vi "Single Shimmer.vi"() -> ()   [LabVIEW 2025]
uses:
  C:/Github/Shimmer-Labview-API/ShimmerLabview/Bin/ShimmerLVWrapper.dll
  Bin/ShimmerLVWrapper.dll
panel:
  out "Waveform Chart":cluster{dbl, dbl, dbl}(graph)
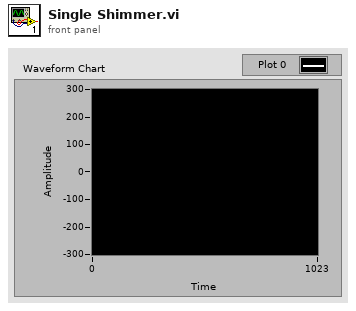
[diagram p1: front panel]
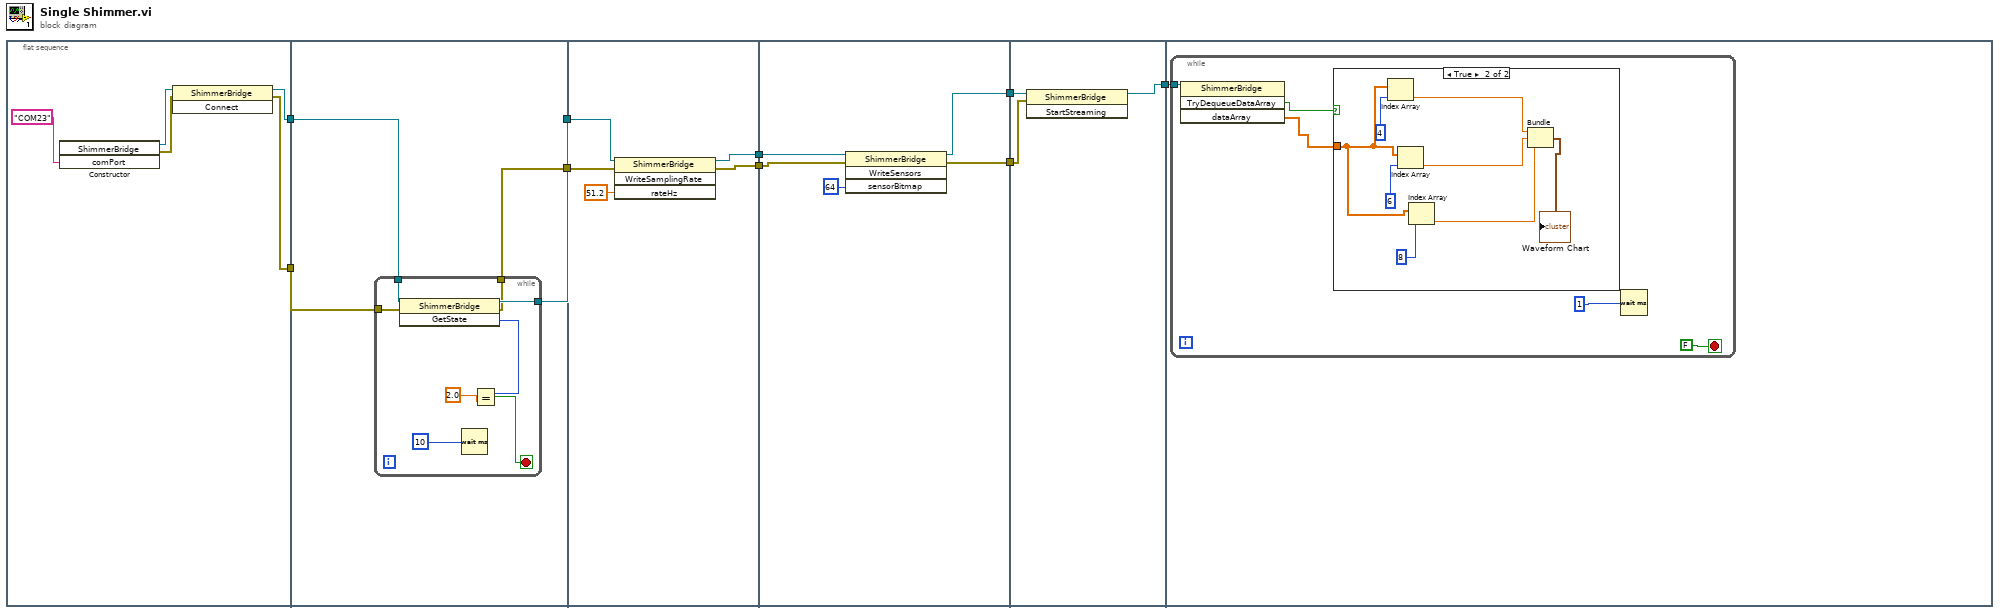
[diagram p0: block diagram]
diagram:
  n1 = flat-sequence {
    tunnel: [w11] -> w9
    tunnel: [w10] -> w4
    tunnel: w9 -> [w18]
    tunnel: [w17] -> w7
    tunnel: w4 -> [w15]
    tunnel: [w16] -> w1
    tunnel: w7 -> [w31]
    tunnel: [w30] -> w6
    tunnel: [w29] -> w3
    tunnel: w1 -> [w27]
    tunnel: w6 -> [w36]
    tunnel: [w35] -> w5
    tunnel: w3 -> [w34]
    tunnel: [w33] -> w2
    tunnel: [w39] -> w8
    tunnel: w5 -> [w38]
    tunnel: w2 -> [w37]
    tunnel: w8 -> [w40]
    frame #0 {
      n2 = constructor class="ShimmerBridge"("comPort"="COM23") -> (reference out=w13:refnum<k24>, error out=w12:errorcluster)  [unwired: 3 in, 2 out]
      n3 = invoke class="ShimmerBridge" method="Connect"(reference=w13, error in=w12) -> (reference out=w11:refnum<k24>, error out=w10:errorcluster)  [unwired: 1 in, 1 out]
    }
    frame #1 {
      n4 = while {
        tunnel: w18 -> [w24]
        tunnel: [w23] -> w17
        tunnel: [w22] -> w16
        tunnel: w15 -> [w21]
        stop <- w26 stop-if-true
        n5 = invoke class="ShimmerBridge" method="GetState"(reference=w24, error in=w21) -> (reference out=w23:refnum<k24>, error out=w22:errorcluster, "GetState"=w20:i32)  [unwired: 1 in]
        n6 = Wait (ms)(milliseconds to wait=u32 10 ("millisecond timer value")) -> ()  [unwired: 1 out]
        n7 = Equal?(x=w20, y=2.0 ("rateHz")) -> (x = y?=w26:bool)
      }
    }
    frame #2 {
      n8 = invoke class="ShimmerBridge" method="WriteSamplingRate"(reference=w31, error in=w27, "rateHz"=51.2) -> (reference out=w30:refnum<k24>, error out=w29:errorcluster)  [unwired: 1 in, 2 out]
    }
    frame #3 {
      n9 = invoke class="ShimmerBridge" method="WriteSensors"(reference=w36, error in=w34, "sensorBitmap"=64) -> (reference out=w35:refnum<k24>, error out=w33:errorcluster)  [unwired: 1 in, 2 out]
    }
    frame #4 {
      n10 = invoke class="ShimmerBridge" method="StartStreaming"(reference=w38, error in=w37) -> (reference out=w39:refnum<k24>)  [unwired: 1 in, 2 out]
    }
    frame #5 {
      n11 = while {
        tunnel: w40 -> [w43]
        stop <- FALSE stop-if-true
        n12 = invoke class="ShimmerBridge" method="TryDequeueDataArray"(reference=w43) -> ("TryDequeueDataArray"=w42:bool, "dataArray"=w41:dbl[])  [unwired: 3 in, 2 out]
        n13 = case shown="True" w42 {
          tunnel: w41 -> [_ w50]
          frame False {
          }
          frame True {
            n14 = Index Array(array=w50, index=4) -> (element=w49:dbl)
            n15 = Index Array(array=w50, index=6) -> (element=w48:dbl)
            n16 = Index Array(array=w50, index=8) -> (element=w47:dbl)
            n17 = Bundle(w49, w48, w47) -> (→"Waveform Chart":cluster{dbl, dbl, dbl})  [unwired: 1 in]
          }
        }
        n18 = Wait (ms)(milliseconds to wait=u32 1) -> ()  [unwired: 1 out]
      }
    }
  }
